vi "ClassExample.vi"() -> ()   [LabVIEW 2025]
panel:
  out "Array 3":bool[](array[boolean])
  out "size(s)":i32
  in  "Array 2":dbl[](array[numeric])
  out "Array":dbl[](array[numeric])
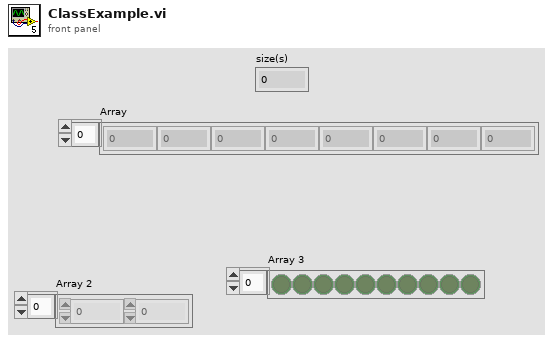
[diagram p1: front panel]
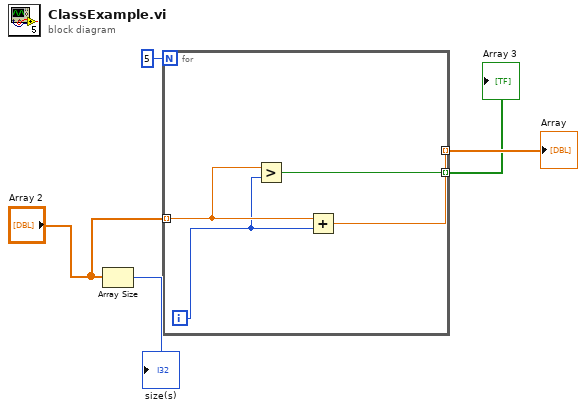
[diagram p0: block diagram]
diagram:
  n1 = Array Size(array="Array 2") -> (size(s)=→"size(s)":i32)
  n2 = for {
    N: 5 -> [_]
    tunnel: [w9] -> w5 mode=indexing
    tunnel: "Array 2" -> [w8] mode=indexing
    tunnel: [w6] -> w1 mode=indexing
    i -> [w7]
    n3 = Greater?(x=w8, y=w7) -> (0:w6:bool)
    n4 = Add(x=w8, y=w7) -> (x+y=w9:dbl)
  }
  "Array" <- w5
  "Array 3" <- w1
